vi "SerialDevice.vi"(4 "error in (no error)":errorcluster, 5 "Out":refnum<k21>, 6 "In":refnum<k21>, 7 "Port":refnum<k21>) -> (0 "error out":errorcluster)   [LabVIEW 2023]
uses:
  <vilib>/rvi/Emulation/niFpgaGetClockAttributes.vi
  <vilib>/rvi/Emulation/niFpgaSctlEmulationGetInTimedLoop.vi
  <vilib>/rvi/Emulation/niFpgaEmulationReportErrorSimple.vi
  <vilib>/rvi/Emulation/niFpgaProcessEmulError.vi
  <vilib>/rvi/DataTransferAndStorage/Container/Common/niFpgaContainerGetUniqueNameForEmu.vi
  <vilib>/rvi/DataTransferAndStorage/Container/Common/niFpgaContainerSetEmuInfo.vi
  <vilib>/rvi/eio/common/nirviEmuReportErrorAndStop.vi
  <vilib>/rvi/eio/common/nirviEmuTemplateMethod_errors.vi
  <vilib>/rvi/DataTransferAndStorage/Container/Common/niFpgaContainerExecOnDevCompGetState.vi
  <vilib>/rvi/Emulation/niFpgaEmulationIsFPGAContextNoSignature.vi
  <vilib>/rvi/errors/niFpgaSetErrorForExecOnDevCompSimple.vi
  <vilib>/rvi/FIFO/Fifo_Resource/nirvififoEmulationSetSize.vi
  <vilib>/rvi/FIFO/Fifo_Resource/nirviFifoEmulationQueueMgr.vi
  <instcachedir>/0/nirviFifoEmulationQueueMgr_E5CAEC123FF24DC58D834DCA3CDAA9B5.lvgen/nirviFifoEmulationQueueMgr_E5CAEC123FF24DC58D834DCA3CDAA9B5_002.vi
  <vilib>/rvi/FIFO/Fifo_Resource/nirvififoEmulationDetermineInputValidOut.vi
  <vilib>/rvi/FIFO/Fifo_Resource/nirvififoEmulationCreateLock.vi
  <vilib>/rvi/FIFO/Fifo_Resource/nirvififoEmulationObtainLock.vi
  <vilib>/rvi/FIFO/Fifo_Resource/nirvififoEmulationReleaseLock.vi
  <vilib>/rvi/occurrence/nirviWaitOnOccurrenceBase.vi
  <vilib>/rvi/errors/nirviReportUnexpectedCaseInternalError.vi
  <vilib>/rvi/errors/nirviReportUnexpectedCaseInternalError (U32).vi
  <vilib>/Utility/error.llb/Clear Errors.vi
  <vilib>/eio/utilities/niEioResolveVilibRelativePath.vi
  <vilib>/rvi/interface/RandomDataEmulation/niFpgaRandomDataHandleErrors.vi
  <vilib>/rvi/Emulation/niFpgaCriticalErrorInLSC.vi
  <vilib>/rvi/LocalResourceManager/LocalResourceManager.xnode
  <vilib>/eio/EIOMethodNode/EIOMethodNode.xnode
  <vilib>/rvi/DataTransferAndStorage/Container/XNode/niFpgaContainer.xnode
  <vilib>/rvi/FIFO/Fifo_Resource/niFpgaFifoEmulationRefIn.vi
panel:
  out "Timeouted":bool
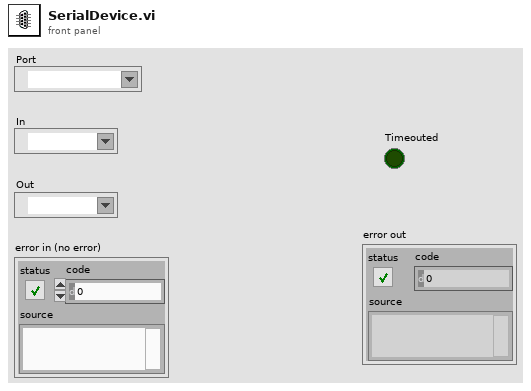
[diagram p1: front panel]
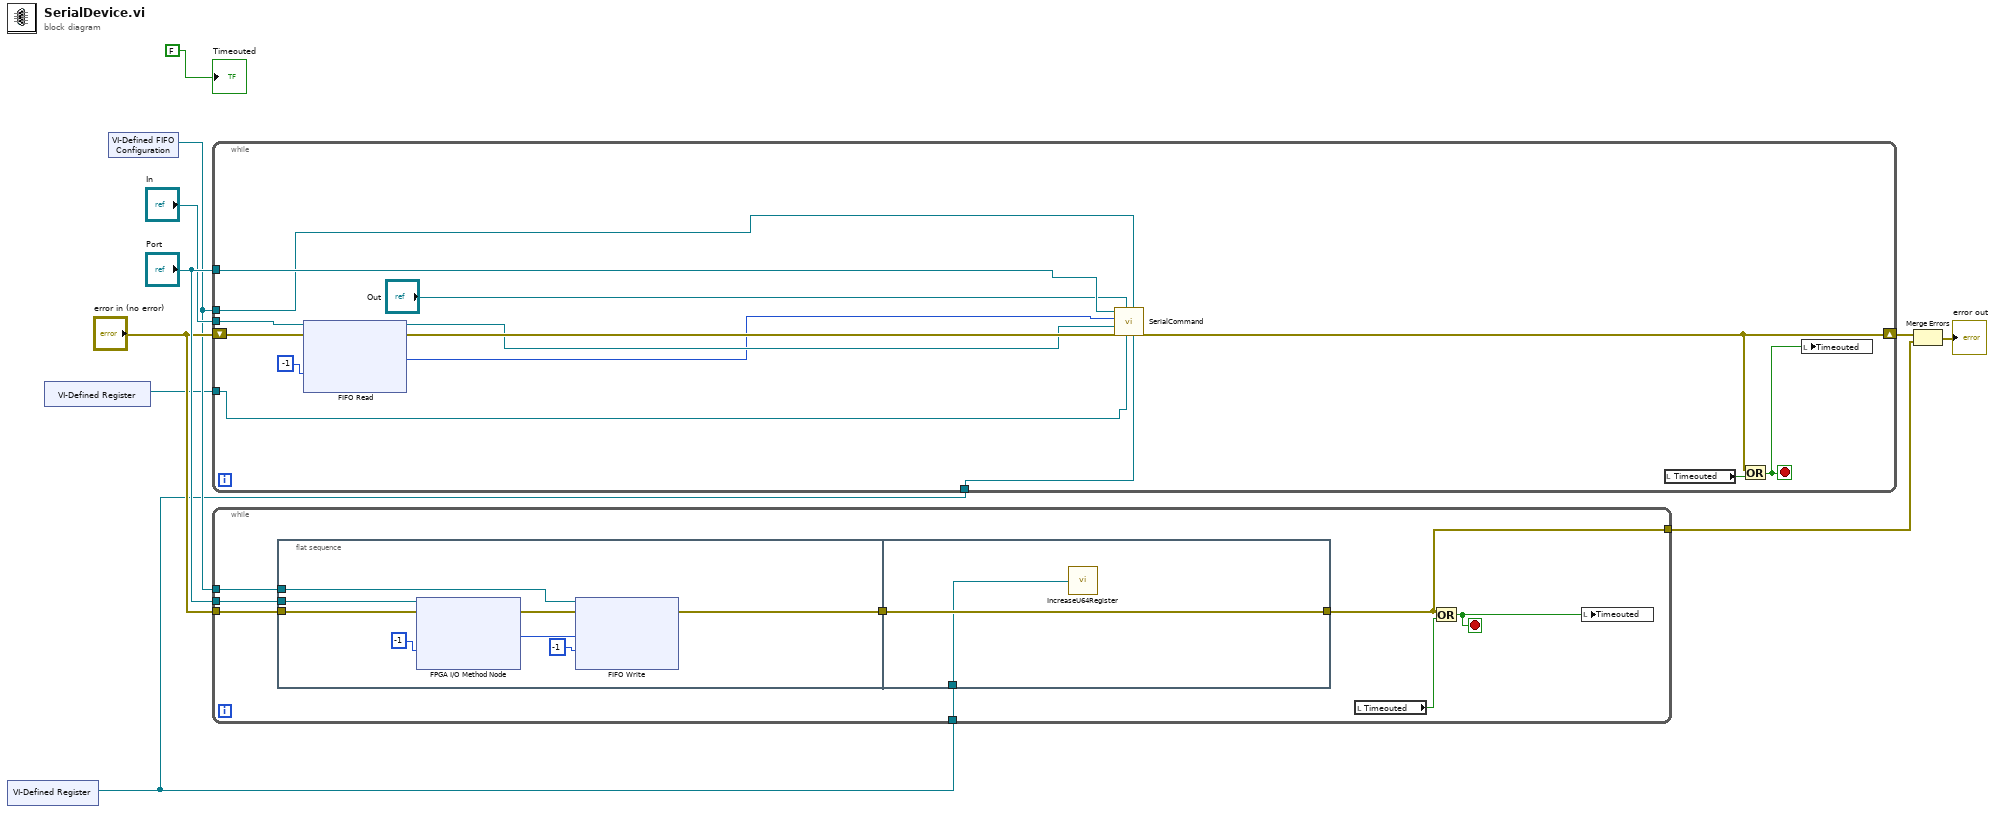
[diagram p0: block diagram]
diagram:
  n1 = xnode "VI-Defined Register"() -> ("Register Out"=w2:refnum<k21>)
  n2 = xnode "VI-Defined Register"() -> ("Register Out"=w1:refnum<k21>)
  n3 = xnode "VI-Defined FIFO Configuration"() -> ("FIFO Out"=w4:refnum<k21>)
  n4 = while {
    tunnel: "Port" -> [w24]
    tunnel: "In" -> [w23]
    shift-right: [w19] -> w7
    shift-left: "error in (no error)" -> [w22]
    tunnel: w4 -> [w13]
    tunnel: w2 -> [w16]
    tunnel: w1 -> [w11]
    stop <- w18 stop-if-true
    n5 = xnode ("FIFO Read")("Timeout"=-1, "error in (no error)"=w22, "FIFO In"=w23) -> ("Element"=w14:u8, "error out"=w21:errorcluster, "FIFO Out"=w15:refnum<k21>)  [unwired: 1 out]
    n6 = call "SerialCommand.vi"("Received"=w16, "ReceivedBuffer"=w13, "Transmitted"=w11, "Out"="Out", "error in (no error)"=w21, "CommandFIFO"=w15, "Command"=w14, "Port"=w24) -> ("error out"=w19:errorcluster)  [unwired: 3 in]
    n7 = local read "Timeouted"() -> (w17:bool)
    n8 = Or(x=w19, y=w17) -> (x .or. y?=w18:bool)
    n9 = local write "Timeouted"(w18) -> ()
  }
  n10 = while {
    tunnel: w4 -> [w32]
    tunnel: "Port" -> [w31]
    tunnel: "error in (no error)" -> [w30]
    tunnel: [w28] -> w8
    tunnel: w2 -> [w25]
    stop <- w27 stop-if-true
    n11 = flat-sequence {
      tunnel: [w33] -> w29
      tunnel: w32 -> [w40]
      tunnel: w31 -> [w38]
      tunnel: w30 -> [w35]
      tunnel: [w42] -> w28
      tunnel: w29 -> [w42]
      tunnel: w25 -> [w41]
      frame #0 {
        n12 = xnode "FPGA I/O Method Node"("error in"=w35, "FPGA I/O In"=w38, "Timeout (ms)"=-1) -> ("error out"=w34:errorcluster, "Data"=w37:u8)  [unwired: 2 out]
        n13 = xnode ("FIFO Write")("Element"=w37, "Timeout"=-1, "error in (no error)"=w34, "FIFO In"=w40) -> ("error out"=w33:errorcluster)  [unwired: 2 out]
      }
      frame #1 {
        n14 = call "IncreaseU64Register.vi"("Register In"=w41) -> ()  [unwired: 1 out]
      }
    }
    n15 = local read "Timeouted"() -> (w26:bool)
    n16 = Or(x=w28, y=w26) -> (x .or. y?=w27:bool)
    n17 = local write "Timeouted"(w27) -> ()
  }
  n18 = Merge Errors(w7, w8) -> (→"error out":errorcluster)
  "Timeouted" <- FALSE ("Boolean")
